vi "Write Xscale_range.vi"(8 "error in (no error)":errorcluster, 10 "Xscale_range":cluster{"start pixel":dbl, "stop_pixel":dbl}, 11 "Detector in":refnum<class "Detector.lvclass">) -> (0 "error out":errorcluster, 3 "Detector out":refnum<class "Detector.lvclass">)   [LabVIEW 2020, in "Detector.lvclass"]
uses:
  Detector.lvclass
  Detector.lvclass/Detector.ctl
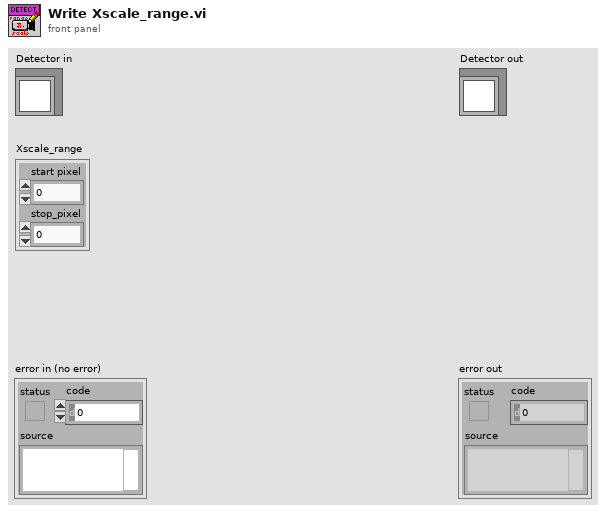
[diagram p1: front panel]
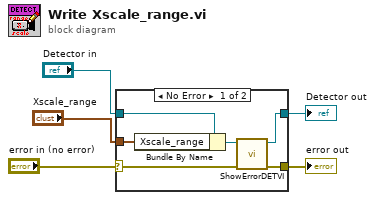
[diagram p0: block diagram]
diagram:
  n1 = case shown="No Error" "error in (no error)" {
    selector: "error in (no error)" -> [w8 w12]
    tunnel: [w7 w12] -> w4
    tunnel: [w6 w13] -> w2
    tunnel: "Detector in" -> [w11 w13]
    tunnel: "Xscale_range" -> [w10 _]
    frame No Error {
      n2 = Bundle By Name(cluster=w11, "Xscale_range"=w10) -> (w9:refnum<class "Detector.lvclass">)
      n3 = call "ShowErrorDETVI.vi"("error in (no error)"=w8, "Detector in"=w9) -> ("error out"=w7:errorcluster, "Detector out"=w6:refnum<class "Detector.lvclass">)  [unwired: 8 in]
    }
    frame Error {
    }
  }
  "error out" <- w4
  "Detector out" <- w2
